vi "Xml_Load_Experiment.vi"(7 "Version String":string, 8 "error in (no error)":errorcluster, 10 "XML Path":path=path "D:/TEST.xml", 11 "Refnum Clust":refnum<vi>) -> (0 "error out":errorcluster)   [LabVIEW 2018]
uses:
  controls/EXPERIMENT_Inputs.ctl
  controls/LASER_Inputs.ctl
  controls/LAMP_Inputs.ctl
  controls/GAS_Inputs.ctl
panel:
  in  "EXPERIMENT Inputs":T1={"Setup"="", "Date"="", "User Name"="", "Comment"="", "Experiment Procedures"=[], "Chemical Source"="", "Sample Components"=[], "Species"=[], "Laser 1"={"Used"=TRUE, "Name"="Spectroscopy", "Wavelength"=1000.0, "Energy"=25.0}, "Laser 2"={"Used"=TRUE, "Name"="Spectroscopy", "Wavelength"=1000.0, "Energy"=25.0}, "Laser 3"={"Used"=TRUE, "Name"="Spectroscopy", "Wavelength"=1000.0, "Energy"=25.0}, "Laser 4"={"Used"=TRUE, "Name"="Spectroscopy", "Wavelength"=1000.0, "Energy"=25.0}, "Laser 5"={"Used"=TRUE, "Name"="Spectroscopy", "Wavelength"=1000.0, "Energy"=25.0}, "Lamp 1"={"Used"=TRUE, "Name"="Spectroscopy", "Wavelength"=1000.0, "Attenuation"=25.0}, "Lamp 2"={"Used"=TRUE, "Name"="Spectroscopy", "Wavelength"=1000.0, "Attenuation"=25.0}, "Gas 1"={"Used"=TRUE, "Name"="Spectroscopy", "Pressure"=1000.0}, "Gas 2"={"Used"=TRUE, "Name"="Spectroscopy", "Pressure"=1000.0}, "Gas 3"={"Used"=TRUE, "Name"="Spectroscopy", "Pressure"=1000.0}, "Gas 4"={"Used"=TRUE, "Name"="Spectroscopy", "Pressure"=1000.0}, "Gas 5"={"Used"=TRUE, "Name"="Spectroscopy", "Pressure"=1000.0}}
  # "Lasers"
  # "nm"
  # "mJ"
  # "Lamps"
  # "nm"
  # "dB"
  # "Gas"
  # "bar"
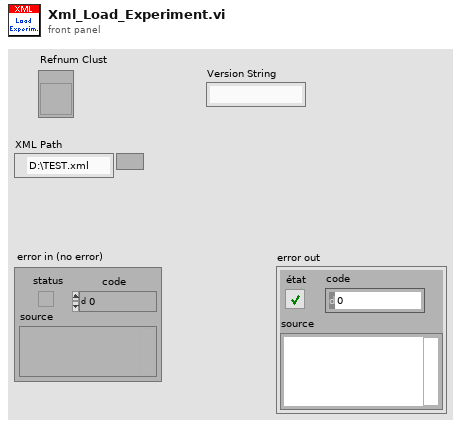
[diagram p1: front panel]
types:
  T1 = typedef "EXPERIMENT_Inputs.ctl" = cluster{"Setup":string, "Date":string, "User Name":string, "Comment":string, "Experiment Procedures":string[], "Chemical Source":string, "Sample Components":string[], "Species":string[], "Laser 1":T2, "Laser 2":T2, "Laser 3":T2, "Laser 4":T2, "Laser 5":T2, "Lamp 1":T3, "Lamp 2":T3, "Gas 1":T4, "Gas 2":T4, "Gas 3":T4, "Gas 4":T4, "Gas 5":T4}
  T2 = typedef "LASER_Inputs.ctl" = cluster{"Used":bool, "Name":string, "Wavelength":dbl, "Energy":dbl}
  T3 = typedef "LAMP_Inputs.ctl" = cluster{"Used":bool, "Name":string, "Wavelength":dbl, "Attenuation":dbl}
  T4 = typedef "GAS_Inputs.ctl" = cluster{"Used":bool, "Name":string, "Pressure":dbl}
  T5 = cluster{"Setup":string, "Date":string, "User Name":string, "Comment":string, "Experiment Procedures":string[], "Chemical Source":string, "Sample Components":string[], "Species":string[], "Laser 1":T2, "Laser 2":T2, "Laser 3":T2, "Laser 4":T2, "Laser 5":T2, "Gas":string[]}
  T6 = cluster{"User Name":string, "Date":string, "Comment":string, "Experiment Steps":string[], "Sample Components":string[], "Molecules":string[], "Laser 1":T2, "Laser 2":T2, "Laser 3":T2}
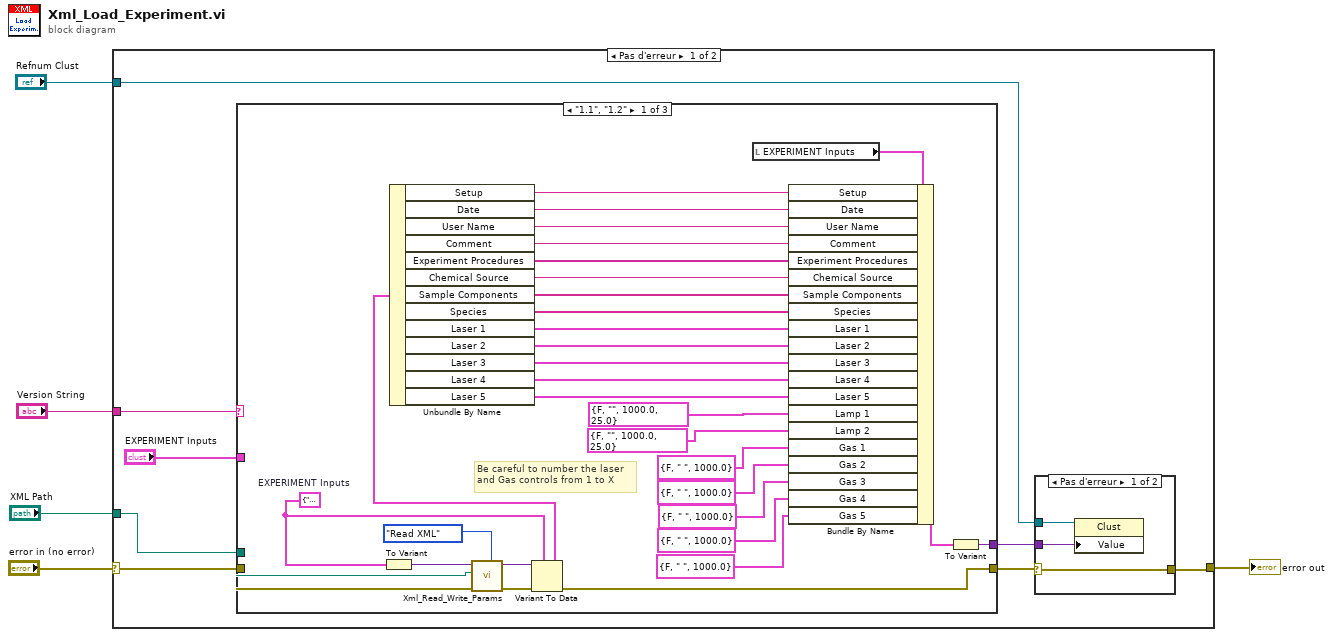
[diagram p0: block diagram]
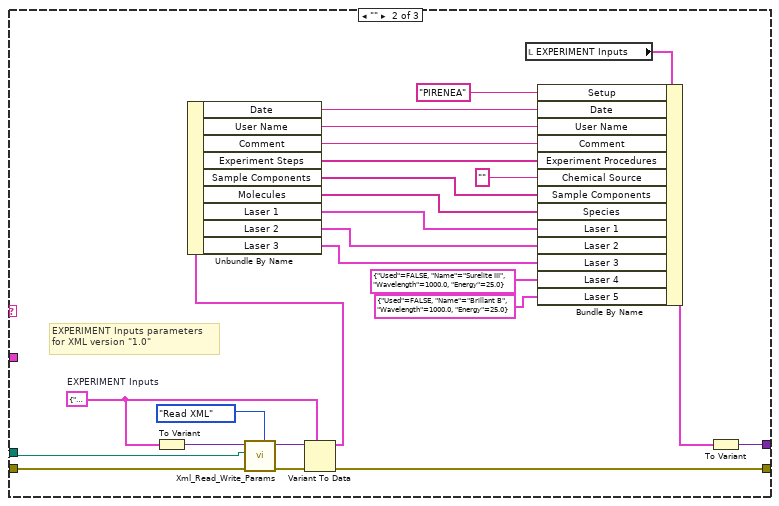
[diagram p2: hidden frame]
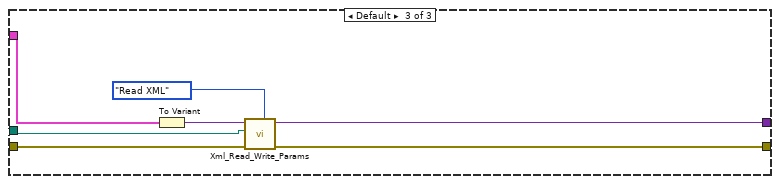
[diagram p3: hidden frame]
diagram:
  n1 = case shown="Pas d'erreur" "error in (no error)" {
    selector: "error in (no error)" -> [w13 w82]
    tunnel: [w9 w82] -> w1
    tunnel: "XML Path" -> [w12 _]
    tunnel: "Version String" -> [w11 _]
    tunnel: "Refnum Clust" -> [w7 _]
    frame No Error {
      n2 = case shown="\"1.1\", \"1.2\"" w11 {
        tunnel: w13 -> [w43 w68 w75]
        tunnel: [w32 w49 w73] -> w10
        tunnel: [w34 w51 w74] -> w8
        tunnel: w12 -> [w41 w66 w72]
        tunnel: "EXPERIMENT Inputs" -> [_ _ w71]
        frame "1.1", "1.2" {
          w30 = T5 {"Setup"="", "Date"="", "User Name"="", "Comment"="", "Experiment Procedures"=[], "Chemical Source"="", "Sample Components"=[], "Species"=[], "Laser 1"={"Used"=TRUE, "Name"="Spectroscopy", "Wavelength"=1000.0, "Energy"=25.0}, "Laser 2"={"Used"=TRUE, "Name"="Spectroscopy", "Wavelength"=1000.0, "Energy"=25.0}, "Laser 3"={"Used"=TRUE, "Name"="Spectroscopy", "Wavelength"=1000.0, "Energy"=25.0}, "Laser 4"={"Used"=TRUE, "Name"="Spectroscopy", "Wavelength"=1000.0, "Energy"=25.0}, "Laser 5"={"Used"=TRUE, "Name"="Spectroscopy", "Wavelength"=1000.0, "Energy"=25.0}, "Gas"=[]}  # EXPERIMENT Inputs
          # "Be careful to number the laser\nand Gas controls from 1 to X"
          n3 = To Variant(anything=w30) -> (Variant=w44:variant)
          n4 = call "Xml_Read_Write_Params.vi"("Variant"=w44, "XML Path"=w41, "error in (no error)"=w43, "Command"=enum16{"Read XML", "Set", "Get", "Write XML"}."Read XML") -> ("Variant Output"=w42:variant, "error out"=w40:errorcluster)  [unwired: 3 in, 1 out]
          n5 = Variant To Data(error in=w40, type=w30, Variant=w42) -> (data=w39:T5, error out=w32:errorcluster)
          n6 = Unbundle By Name(w39) -> ("Setup"=w29:string, "Date"=w28:string, "User Name"=w27:string, "Comment"=w26:string, "Experiment Procedures"=w25:string[], "Chemical Source"=w24:string, "Sample Components"=w23:string[], "Species"=w22:string[], "Laser 1"=w35:T2, "Laser 2"=w36:T2, "Laser 3"=w37:T2, "Laser 4"=w21:T2, "Laser 5"=w20:T2)
          n7 = local read "EXPERIMENT Inputs"() -> (w38:T1)
          n8 = Bundle By Name(cluster=w38, "Setup"=w29, "Date"=w28, "User Name"=w27, "Comment"=w26, "Experiment Procedures"=w25, "Chemical Source"=w24, "Sample Components"=w23, "Species"=w22, "Laser 1"=w35, "Laser 2"=w36, "Laser 3"=w37, "Laser 4"=w21, "Laser 5"=w20, "Lamp 1"=T3 {"Used"=FALSE, "Name"="", "Wavelength"=1000.0, "Attenuation"=25.0}, "Lamp 2"=T3 {"Used"=FALSE, "Name"="", "Wavelength"=1000.0, "Attenuation"=25.0}, "Gas 1"=T4 {"Used"=FALSE, "Name"=" ", "Pressure"=1000.0}, "Gas 2"=T4 {"Used"=FALSE, "Name"=" ", "Pressure"=1000.0}, "Gas 3"=T4 {"Used"=FALSE, "Name"=" ", "Pressure"=1000.0}, "Gas 4"=T4 {"Used"=FALSE, "Name"=" ", "Pressure"=1000.0}, "Gas 5"=T4 {"Used"=FALSE, "Name"=" ", "Pressure"=1000.0}) -> (w33:T1)
          n9 = To Variant(anything=w33) -> (Variant=w34:variant)
        }
        frame "" {
          w64 = T6 {"User Name"="", "Date"="", "Comment"="", "Experiment Steps"=[], "Sample Components"=[], "Molecules"=[], "Laser 1"={"Used"=TRUE, "Name"="Spectroscopy", "Wavelength"=1000.0, "Energy"=25.0}, "Laser 2"={"Used"=TRUE, "Name"="Spectroscopy", "Wavelength"=1000.0, "Energy"=25.0}, "Laser 3"={"Used"=TRUE, "Name"="Spectroscopy", "Wavelength"=1000.0, "Energy"=25.0}}  # EXPERIMENT Inputs
          # "EXPERIMENT Inputs parameters\nfor XML version \"1.0\""
          n10 = To Variant(anything=w64) -> (Variant=w69:variant)
          n11 = call "Xml_Read_Write_Params.vi"("Variant"=w69, "XML Path"=w66, "error in (no error)"=w68, "Command"=enum16{"Read XML", "Set", "Get", "Write XML"}."Read XML") -> ("Variant Output"=w67:variant, "error out"=w65:errorcluster)  [unwired: 3 in, 1 out]
          n12 = Variant To Data(error in=w65, type=w64, Variant=w67) -> (data=w63:T6, error out=w49:errorcluster)
          n13 = Unbundle By Name(w63) -> ("Date"=w61:string, "User Name"=w60:string, "Comment"=w59:string, "Experiment Steps"=w58:string[], "Sample Components"=w57:string[], "Molecules"=w56:string[], "Laser 1"=w54:T2, "Laser 2"=w55:T2, "Laser 3"=w48:T2)
          n14 = local read "EXPERIMENT Inputs"() -> (w62:T1)
          n15 = Bundle By Name(cluster=w62, "Setup"="PIRENEA", "Date"=w61, "User Name"=w60, "Comment"=w59, "Experiment Procedures"=w58, "Chemical Source"="", "Sample Components"=w57, "Species"=w56, "Laser 1"=w54, "Laser 2"=w55, "Laser 3"=w48, "Laser 4"=T2 {"Used"=FALSE, "Name"="Surelite III", "Wavelength"=1000.0, "Energy"=25.0}, "Laser 5"=T2 {"Used"=FALSE, "Name"="Brillant B", "Wavelength"=1000.0, "Energy"=25.0}) -> (w50:T1)
          n16 = To Variant(anything=w50) -> (Variant=w51:variant)
        }
        frame Default {
          n17 = To Variant(anything=w71) -> (Variant=w76:variant)
          n18 = call "Xml_Read_Write_Params.vi"("Variant"=w76, "XML Path"=w72, "error in (no error)"=w75, "Command"=enum16{"Read XML", "Set", "Get", "Write XML"}."Read XML") -> ("Variant Output"=w74:variant, "error out"=w73:errorcluster)  [unwired: 3 in, 1 out]
        }
      }
      n19 = case shown="Pas d'erreur" w10 {
        selector: w10 -> [w80 w81]
        tunnel: [w80 w81] -> w9
        tunnel: w8 -> [w79 _]
        tunnel: w7 -> [w78 _]
        frame No Error {
          n20 = property class="Clust"(reference=w78, "Value"=w79) -> ()  [unwired: 1 in, 2 out]
        }
        frame Error {
        }
      }
    }
    frame Error {
    }
  }
  "error out" <- w1
